vi "Untitled ms (SubVI).vi"(10 "time_1":u32, 11 "millisecond timer value":u32) -> (3 "Boolean":bool)   [LabVIEW 2015]
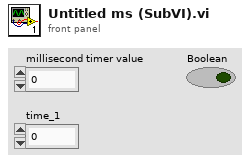
[diagram p1: front panel]
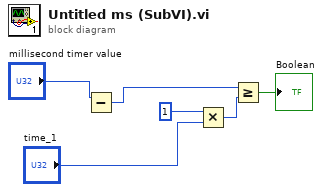
[diagram p0: block diagram]
diagram:
  n1 = Subtract(x="millisecond timer value") -> (x-y=w4:u32)  [unwired: 1 in]
  n2 = Multiply(x=u32 1 ("y"), y="time_1") -> (x*y=w1:u32)
  n3 = Greater Or Equal?(x=w4, y=w1) -> (x >= y?=→"Boolean":bool)
